vi "版本信息解析.vi"(0 "body":string) -> (14 "版本信息":cluster{"版本号":string, "更新内容":string}[](array[cluster]))   [LabVIEW 2016, in "update.lvlib" / "http client.lvclass"]
uses:
  http client.lvclass
  <vilib>/regexp/Match Regular Expression.xnode
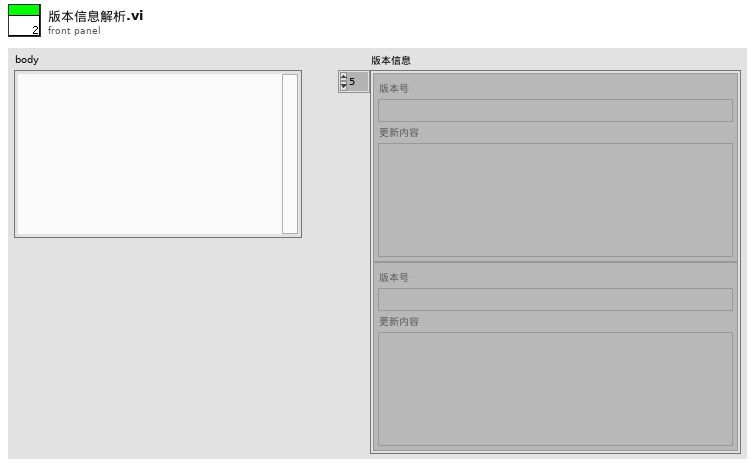
[diagram p1: front panel]
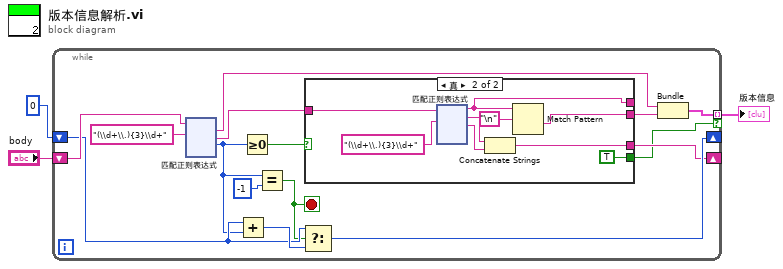
[diagram p0: block diagram]
diagram:
  n1 = while {
    shift-right: [w8] -> _
    shift-left: "body" -> [w17]
    shift-right: [w16] -> _
    shift-left: 0 ("匹配后偏移量") -> [w14]
    tunnel: [w6] -> w1 mode=indexing if=w5
    stop <- w12 stop-if-true
    n2 = xnode "匹配正则表达式"("输入字符串"=w17, "正则表达式"="(\\d+\\.){3}\\d+") -> ("所有匹配"=w7:string, "匹配之后"=w9:string, "匹配后偏移量"=w11:i32)  [unwired: 4 in, 2 out]
    n3 = Add(x=w14, y=w11) -> (x+y=w15:i32)
    n4 = Greater Or Equal To 0?(x=w11) -> (x >= 0?=w10:bool)
    n5 = Equal?(x=w11, y=-1) -> (x = y?=w12:bool)
    n6 = Select(t=w14, s=w12, f=w15) -> (s? t:f=w16:i32)
    n7 = case shown="真" w10 {
      tunnel: w9 -> [w19 w27]
      tunnel: [w19 w24] -> w8
      tunnel: [_ w22] -> _
      tunnel: [_ TRUE] -> w5
      tunnel: [_ w20] -> w4
      frame False {
      }
      frame True {
        n8 = xnode "匹配正则表达式"("输入字符串"=w27, "正则表达式"="(\\d+\\.){3}\\d+") -> ("匹配之前"=w22:string, "所有匹配"=w26:string, "匹配之后"=w25:string)  [unwired: 4 in, 2 out]
        n9 = Concatenate Strings(w26, w25) -> (w24:string)
        n10 = Match Pattern(string=w22, regular expression="\n") -> (after substring=w20:string)  [unwired: 1 in, 3 out]
      }
    }
    n11 = Bundle("所有匹配"=w7, "匹配之前"=w4) -> (w6:cluster{"所有匹配":string, "匹配之前":string})  [unwired: 1 in]
  }
  "版本信息" <- w1
